vi "MeasDetails.vi"(10 "measurement":string, 11 "Configuration In":T1) -> (0 "error out":errorcluster, 3 "Configuration out":T1)   [LabVIEW 2021, in "dcvmDPI_AD7606B_serverImpl.lvlib"]
uses:
  dcvmDPI_AD7606B_serverImpl.lvlib
  controls/configuration.ctl
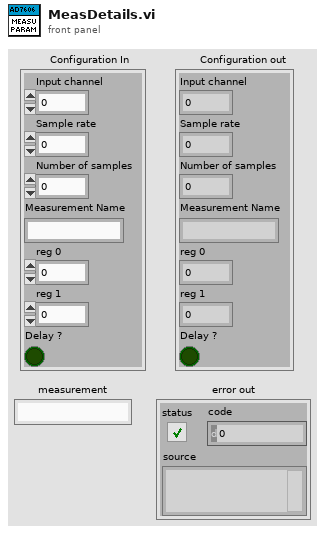
[diagram p1: front panel]
types:
  T1 = typedef "dcvmDPI_AD7606B_serverImpl.lvlib/configuration.ctl" = cluster{"Input channel":i32, "Sample rate":dbl, "Number of samples":u32, "Measurement Name":string, "reg 0":i32, "reg 1":i32, "Delay ?":bool}
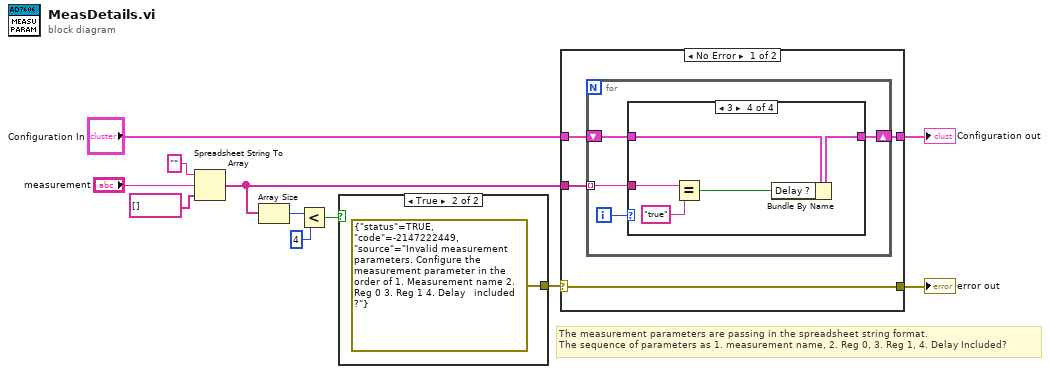
[diagram p0: block diagram]
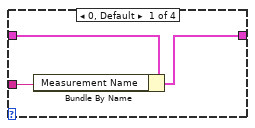
[diagram p2: hidden frame]
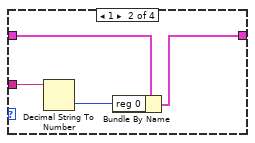
[diagram p3: hidden frame]
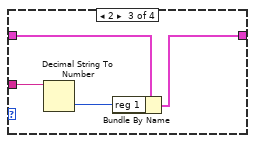
[diagram p4: hidden frame]
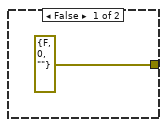
[diagram p6: hidden frame]
diagram:
  # "The measurement parameters are passing in the spreadsheet string format.\nThe sequence of parameters as 1. measurement name, 2. Reg 0, 3. Reg 1, 4. Delay Included?"
  n1 = Spreadsheet String To Array(format string="", spreadsheet string="measurement", array type (2D Dbl)=string[] []) -> (array=w6:string[])  [unwired: 1 in]
  n2 = Array Size(array=w6) -> (size(s)=w5:i32)
  n3 = Less?(x=w5, y=4) -> (x < y?=w3:bool)
  n4 = case shown="True" w3 {
    tunnel: [errorcluster {"status"=FALSE, "code"=0, "source"=""} ("error constant") errorcluster {"status"=TRUE, "code"=-2147222449, "source"="Invalid measurement parameters. Configure the measurement parameter in the order of 1. Measurement name 2. Reg 0 3. Reg 1 4. Delay   included ?"} ("error in")] -> w2
    frame False {
    }
    frame True {
    }
  }
  n5 = case shown="No Error" w2 {
    selector: w2 -> [w14 w39]
    tunnel: "Configuration In" -> [w17 w38]
    tunnel: [w16 w38] -> w7
    tunnel: w6 -> [w15 _]
    tunnel: [w14 w39] -> w1
    frame No Error {
      n6 = for {
        tunnel: w15 -> [w19] mode=indexing
        shift-right: [w18] -> w16
        shift-left: w17 -> [w20]
        i -> [w21]
        n7 = case shown="3" w21 {
          tunnel: w20 -> [w24 w27 w31 w35]
          tunnel: w19 -> [w23 w28 w32 w37]
          tunnel: [w22 w25 w29 w34] -> w18
          frame 0, Default {
            n8 = Bundle By Name(cluster=w24, "Measurement Name"=w23) -> (w22:T1)
          }
          frame 1 {
            n9 = Decimal String To Number(string=w28) -> (number=w26:i32)  [unwired: 2 in, 1 out]
            n10 = Bundle By Name(cluster=w27, "reg 0"=w26) -> (w25:T1)
          }
          frame 2 {
            n11 = Decimal String To Number(string=w32) -> (number=w30:i32)  [unwired: 2 in, 1 out]
            n12 = Bundle By Name(cluster=w31, "reg 1"=w30) -> (w29:T1)
          }
          frame 3 {
            n13 = Equal?(x=w37, y="true") -> (x = y?=w33:bool)
            n14 = Bundle By Name(cluster=w35, "Delay ?"=w33) -> (w34:T1)
          }
        }
      }
    }
    frame Error {
    }
  }
  "Configuration out" <- w7
  "error out" <- w1
